vi "Flush Data to Log File.vi"(8 "error in (no error)":errorcluster, 10 "Data Queue":refnum<queue>, 11 "Logging Configuration":T1 {"Test Parameters"."Allowed Tolerance (%) FS" format="%#_4g"}) -> (0 "error out":errorcluster)   [LabVIEW 2026, in "Processing_Engine.lvlib"]
doc: "Flush the data queue of any pending data and write it to the log file. Close the TDMS file reference."
uses:
  Processing_Engine.lvlib
  Processing Settings.ctl
  controls/Messaging Payloads/Sensor CoreData.ctl
  controls/Messaging Payloads/Sensor CoreData Cluster.ctl
  controls/UI/Units Enum.ctl
  controls/UI/Signal Enum.ctl
  Test Parameters.ctl
  Test Parameters Cluster.ctl
  controls/UI/Measurement Role.ctl
  controls/UI/Test Sequence Context.ctl
  controls/UI/Direction.ctl
  controls/Messaging Payloads/Processed Calibration Points.ctl
  controls/Messaging Payloads/Processed Calibration Point.ctl
  Test Status.ctl
  Settings/Settings.lvlib
  Analysis/Analysis.lvlib
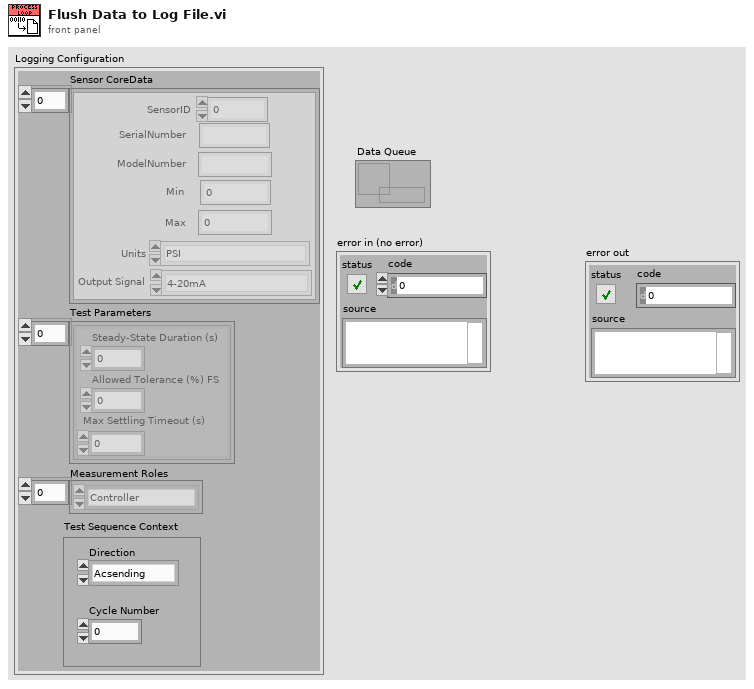
[diagram p1: front panel]
types:
  T1 = typedef "Processing_Engine.lvlib/Processing Settings.ctl" = cluster{"Sensor CoreData":T2, "Test Parameters":T6, "Measurement Roles":T8[], "Test Sequence Context":T9}
  T2 = typedef "Sensor CoreData.ctl" = T3[]
  T3 = typedef "Settings.lvlib/Sensor CoreData Cluster.ctl" = cluster{"SerialNumber":string, "ModelNumber":string, "Min":dbl, "Max":dbl, "Units":T4, "Output Signal":T5, "SensorID":i32}
  T4 = typedef "Units Enum.ctl" = enum16{"PSI", "Deg C", "kPa", "GPM"}
  T5 = typedef "Signal Enum.ctl" = enum16{"4-20mA", "0-10V", "Thermocouple Type K"}
  T6 = typedef "Processing_Engine.lvlib/Test Parameters.ctl" = T7[]
  T7 = typedef "Settings.lvlib/Test Parameters Cluster.ctl" = cluster{"Steady-State Duration (s)":i32, "Allowed Tolerance (%) FS":dbl, "Max Settling Timeout (s)":i32}
  T8 = typedef "Settings.lvlib/Measurement Role.ctl" = enum16{"Controller", "Reference", "UUT", "Disable", "All"}
  T9 = typedef "Settings.lvlib/Test Sequence Context.ctl" = cluster{"Direction":T10, "Cycle Number":i32}
  T10 = typedef "Settings.lvlib/Direction.ctl" = enum16{"Acsending", "Descending"}
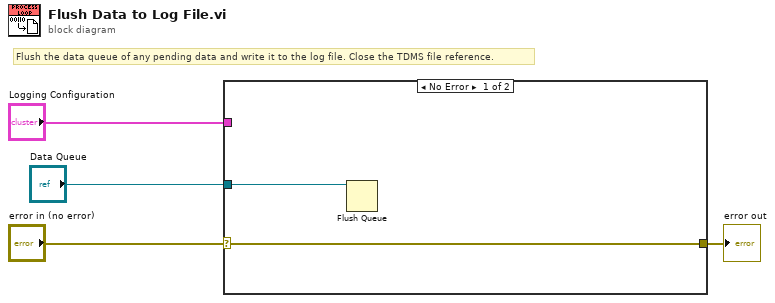
[diagram p0: block diagram]
diagram:
  # "Flush the data queue of any pending data and write it to the log file. Close the TDMS file reference."
  n1 = case shown="No Error" "error in (no error)" {
    selector: "error in (no error)" -> [w5 w7]
    tunnel: "Data Queue" -> [w6 _]
    tunnel: "Logging Configuration" -> [_ _]
    tunnel: [w5 w7] -> w3
    frame No Error {
      n2 = Flush Queue(queue=w6) -> ()  [unwired: 1 in, 3 out]
    }
    frame Error {
    }
  }
  "error out" <- w3
